vi "Create User Event - Stop.vi"(8 "error in (no error)":errorcluster) -> (0 "error out":errorcluster, 3 "User Events":T1)   [LabVIEW 2018, in "GLDL User Event - Stop.lvlib"]
doc: "Create a boolean user event that will be used to stop the event loop from the message handling loop."
uses:
  GLDL User Event - Stop.lvlib
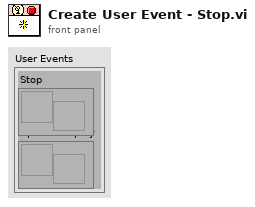
[diagram p1: front panel]
types:
  T1 = cluster{"Stop":refnum<user-event>, "Update Display":refnum<user-event>}
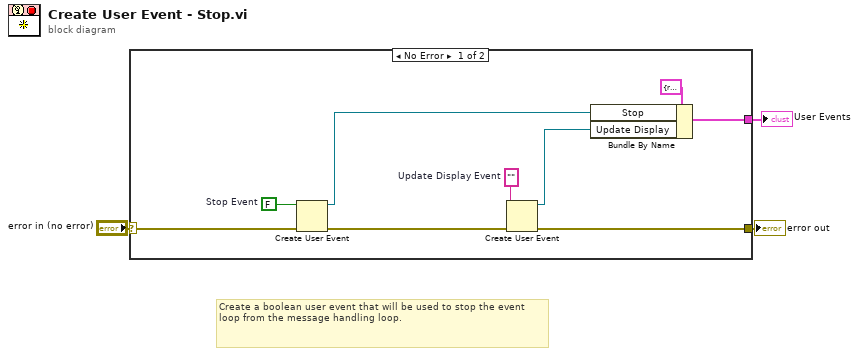
[diagram p0: block diagram]
diagram:
  # "Create a boolean user event that will be used to stop the event loop from the message handling loop."
  n1 = case shown="No Error" "error in (no error)" {
    selector: "error in (no error)" -> [w11 w13]
    tunnel: [w8 w13] -> w3
    tunnel: [w5 _] -> w1
    frame No Error {
      w10 = ""  # Update Display Event
      w12 = FALSE  # Stop Event
      n2 = Create User Event(user event datatype=w12, error in=w11) -> (user event=w7:refnum<user-event>, error out=w9:errorcluster)
      n3 = Create User Event(user event datatype=w10, error in=w9) -> (user event=w6:refnum<user-event>, error out=w8:errorcluster)
      n4 = Bundle By Name(cluster=T1 {"Stop"=refnum, "Update Display"=refnum} ("User Events in"), "Stop"=w7, "Update Display"=w6) -> (w5:T1)
    }
    frame Error {
    }
  }
  "error out" <- w3
  "User Events" <- w1
